vi "AC_6011_INIT.vi"(0 "hDevice(in)":u32, 1 "idd(szin)":u32[](array[numeric])) -> (2 "hDevice(out)":u32, 3 "Cardc":i32, 4 "idd(szout)":u32[](array[numeric]))   [LabVIEW 2015]
uses:
  acpci.dll
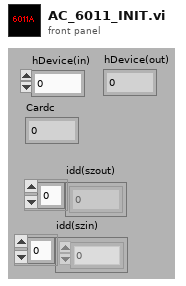
[diagram p1: front panel]
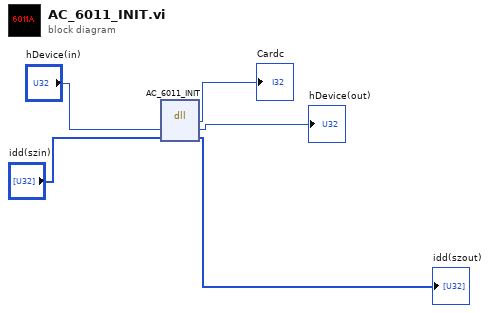
[diagram p0: block diagram]
diagram:
  n1 = dll-call lib="PTH2|abs F2.技术库labviewVI小程序:基于Labview的直流伺服电机位置控制系统设计\t源程序\tACPCI.DLL" fn="AC_6011_INIT"("hDevcie"="hDevice(in)", "idd"="idd(szin)") -> (→"Cardc":i32, "hDevcie"=→"hDevice(out)":u32, "idd"=→"idd(szout)":u32[])  [unwired: 3 in, 2 out]
